vi "log data.vi"(2 "Sensor Data":T1 {"Sensor array"."scaled" format="%.2f"; "Sensor array"."voltage" format="%.4f"; "Time" format="%<%I:%M:%S%2u %p\n%m/%d/%Y>T"}, 3 "refnum":refnum<file>) -> ()   [LabVIEW 2012]
uses:
  TCP DAQ/Sensor data.ctl
  DAQ configuration/sensor cluster.ctl
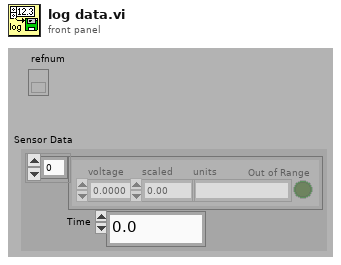
[diagram p1: front panel]
types:
  T1 = typedef "Sensor data.ctl" = cluster{" Sensor array":T2[], "Time":dbl}
  T2 = typedef "sensor cluster.ctl" = cluster{"voltage":sgl, "scaled":sgl, "units":string, "Out of Range":bool}
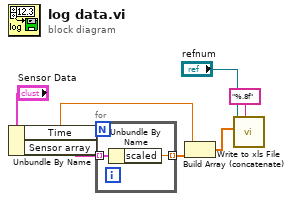
[diagram p0: block diagram]
diagram:
  n1 = Unbundle By Name("Sensor Data") -> ("Time"=w3:dbl, "Sensor array"=w5:T2[])
  n2 = for {
    tunnel: w5 -> [w9] mode=indexing
    tunnel: [w8] -> w4 mode=indexing
    n3 = Unbundle By Name(w9) -> ("scaled"=w8:sgl)
  }
  n4 = Build Array (concatenate)(w3, w4) -> (w1:dbl[])
  n5 = call "Write to xls File.vi"("format (%.3f)"="%.8f", "1D data"=w1, "refnum"="refnum") -> ()  [unwired: 7 in, 2 out]
